vi "2SidedFFT.vi"() -> ()   [LabVIEW 2020]
uses:
  <vilib>/Analysis/2dsp.llb/Real FFT.vi
  <vilib>/Analysis/NI_AALBase.lvlib
  <vilib>/Analysis/NI_AALPro.lvlib
panel:
  out "Spectrum Graph":cluster{i32, dbl, dbl[]}(graph)
  out "Time Domain Sequence":dbl[](graph)
  in  "Sampling Frequency":dbl
  in  "Phase In":dbl
  in  "Signal Frequency":dbl
  in  "No. of Samples":i32
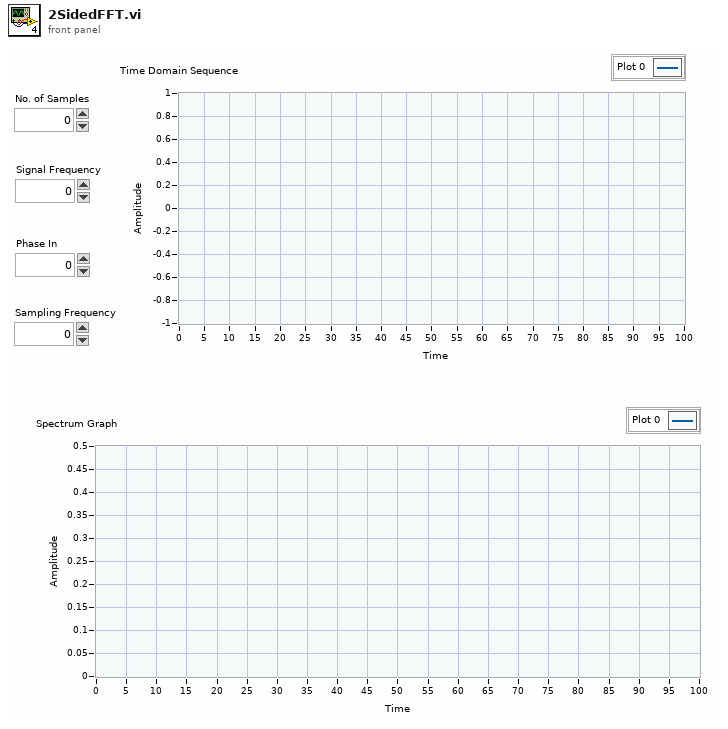
[diagram p1: front panel]
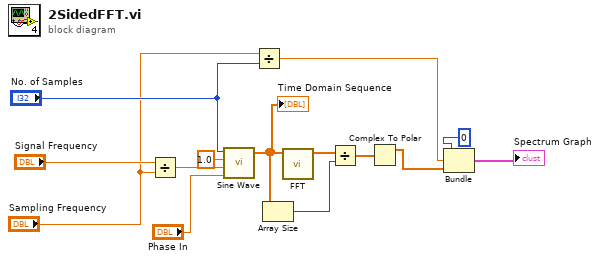
[diagram p0: block diagram]
diagram:
  n1 = Divide(x="Signal Frequency", y="Sampling Frequency") -> (x/y=w13:dbl)
  n2 = call <vilib>:"Sine Wave.vi"("samples"="No. of Samples", "amplitude"=1.0, "frequency"=w13, "phase in"="Phase In") -> ("sine wave"=w2:dbl[])  [unwired: 1 in, 2 out]
  "Time Domain Sequence" <- w2
  n3 = Divide(x="Sampling Frequency", y="No. of Samples") -> (x/y=w5:dbl)
  n4 = Array Size(array=w2) -> (size(s)=w7:i32)
  n5 = call-poly <vilib>:"FFT.vi"("X"=w2) -> ("FFT {X}"=w8:cdb[])  [unwired: 9 in, 1 out]
  n6 = Divide(x=w8, y=w7) -> (x/y=w6:cdb[])
  n7 = Complex To Polar(r * e^(i*theta)=w6) -> (r=w3:dbl[])  [unwired: 1 out]
  n8 = Bundle(0, w5, w3) -> (→"Spectrum Graph":cluster{i32, dbl, dbl[]})  [unwired: 1 in]
